vi "PPS Type Parser.vi"(5 "ClassName":string, 7 "Value":variant, 8 "error in (no error)":errorcluster, 10 "trimmed string":string, 11 "Control in":refnum<vi>) -> (0 "error out":errorcluster, 3 "spreadsheet string":string)   [LabVIEW 2016]
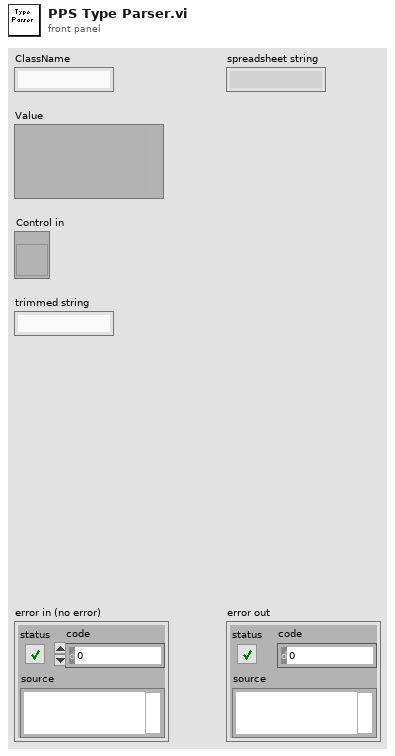
[diagram p1: front panel]
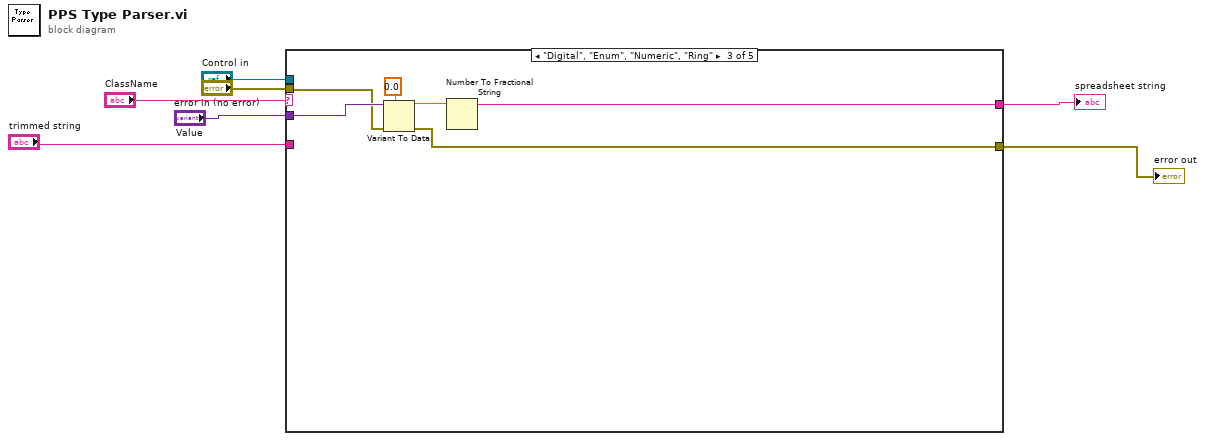
[diagram p0: block diagram]
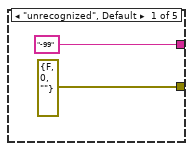
[diagram p2: hidden frame]
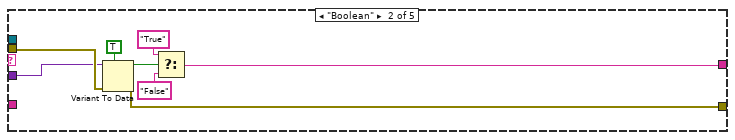
[diagram p3: hidden frame]
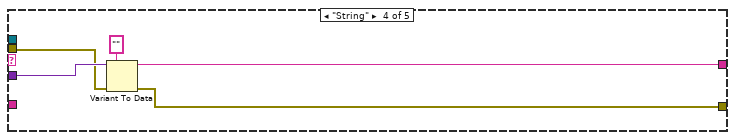
[diagram p4: hidden frame]
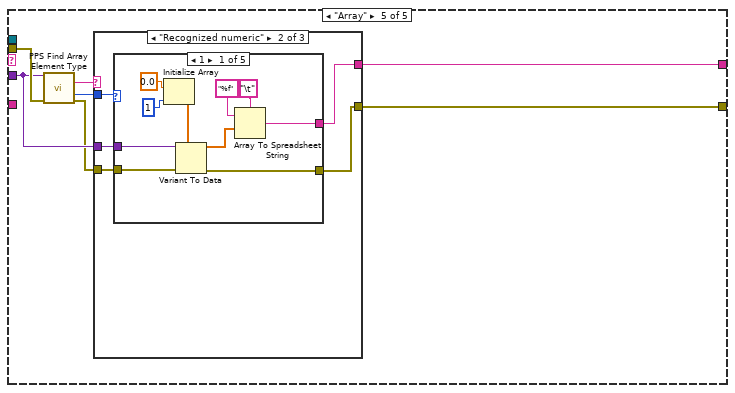
[diagram p5: hidden frame]
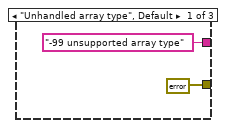
[diagram p6: hidden frame]
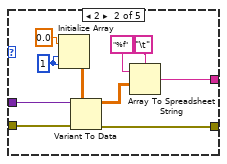
[diagram p7: hidden frame]
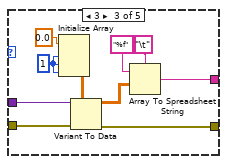
[diagram p8: hidden frame]
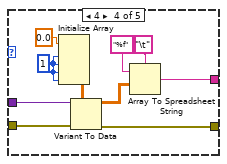
[diagram p9: hidden frame]
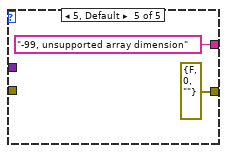
[diagram p10: hidden frame]
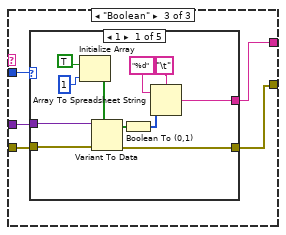
[diagram p11: hidden frame]
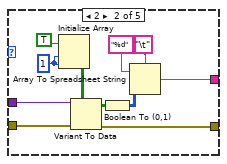
[diagram p12: hidden frame]
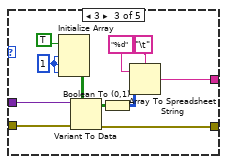
[diagram p13: hidden frame]
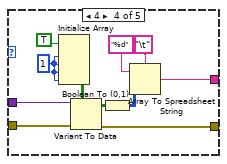
[diagram p14: hidden frame]
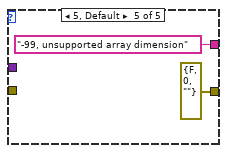
[diagram p15: hidden frame]
diagram:
  n1 = case shown="\"Digital\", \"Enum\", \"Numeric\", \"Ring\"" "ClassName" {
    tunnel: [errorcluster {"status"=FALSE, "code"=0, "source"=""} ("error out") w17 w23 w28 w31] -> w1
    tunnel: "Control in" -> [_ _ _ _ _]
    tunnel: "error in (no error)" -> [_ w11 w18 w24 w35]
    tunnel: ["-99" w12 w21 w27 w32] -> w5
    tunnel: "Value" -> [_ w10 w19 w25 w30]
    tunnel: "trimmed string" -> [_ _ _ _ _]
    frame "unrecognized", Default {
    }
    frame "Boolean" {
      n2 = Variant To Data(error in=w11, type=TRUE, Variant=w10) -> (data=w15:bool, error out=w17:errorcluster)
      n3 = Select(t="True", s=w15, f="False") -> (s? t:f=w12:string)
    }
    frame "Digital", "Enum", "Numeric", "Ring" {
      n4 = Variant To Data(error in=w18, type=0.0, Variant=w19) -> (data=w20:dbl, error out=w23:errorcluster)
      n5 = Number To Fractional String(number=w20) -> (F-format string=w21:string)  [unwired: 3 in]
    }
    frame "String" {
      n6 = Variant To Data(error in=w24, type="" ("data out"), Variant=w25) -> (data=w27:string, error out=w28:errorcluster)
    }
    frame "Array" {
      n7 = call "PPS Find Array Element Type.vi"("Variant"=w30, "error in (no error)"=w35) -> ("Element type Name"=w34:string, "Number of Dimensions"=w33:i32, "error out"=w29:errorcluster)  [unwired: 9 in, 2 out]
      n8 = case shown="\"Recognized numeric\"" w34 {
        tunnel: w33 -> [_ w42 w85]
        tunnel: ["-99 unsupported array type" ("spreadsheet string") w40 w86] -> w32
        tunnel: [errorcluster {"status"=FALSE, "code"=0, "source"=""} ("error out") w38 w87] -> w31
        tunnel: w30 -> [_ w41 w89]
        tunnel: w29 -> [_ w39 w88]
        frame "Unhandled array type", Default {
        }
        frame "Recognized numeric" {
          n9 = case shown="1" w42 {
            tunnel: w41 -> [w47 w58 w68 w78 _]
            tunnel: [w45 w56 w66 w76 "-99, unsupported array dimension" ("spreadsheet string")] -> w40
            tunnel: w39 -> [w44 w55 w65 w75 _]
            tunnel: [w43 w54 w64 w74 errorcluster {"status"=FALSE, "code"=0, "source"=""} ("error out")] -> w38
            frame 1 {
              n10 = Initialize Array(0.0 ("element"), 1 ("dimension size")) -> (w48:dbl[])
              n11 = Variant To Data(error in=w44, type=w48, Variant=w47) -> (data=w46:dbl[], error out=w43:errorcluster)
              n12 = Array To Spreadsheet String(delimiter (Tab)="\t", array=w46, 3:"%f" ("format string")) -> (spreadsheet string=w45:string)
            }
            frame 2 {
              w53 = 1 ("dimension size")
              n13 = Initialize Array(0.0 ("element"), w53, w53) -> (w59:dbl[][])
              n14 = Variant To Data(error in=w55, type=w59, Variant=w58) -> (data=w57:dbl[][], error out=w54:errorcluster)
              n15 = Array To Spreadsheet String(delimiter (Tab)="\t", array=w57, 3:"%f" ("format string")) -> (spreadsheet string=w56:string)
            }
            frame 3 {
              w63 = 1 ("dimension size")
              n16 = Initialize Array(0.0 ("element"), w63, w63, w63) -> (w69:dbl[][][])
              n17 = Variant To Data(error in=w65, type=w69, Variant=w68) -> (data=w67:dbl[][][], error out=w64:errorcluster)
              n18 = Array To Spreadsheet String(delimiter (Tab)="\t", array=w67, 3:"%f" ("format string")) -> (spreadsheet string=w66:string)
            }
            frame 4 {
              w73 = 1 ("dimension size")
              n19 = Initialize Array(0.0 ("element"), w73, w73, w73, w73) -> (w79:dbl[][][][])
              n20 = Variant To Data(error in=w75, type=w79, Variant=w78) -> (data=w77:dbl[][][][], error out=w74:errorcluster)
              n21 = Array To Spreadsheet String(delimiter (Tab)="\t", array=w77, 3:"%f" ("format string")) -> (spreadsheet string=w76:string)
            }
            frame 5, Default {
            }
          }
        }
        frame "Boolean" {
          n22 = case shown="1" w85 {
            tunnel: w89 -> [w96 w108 w119 w130 _]
            tunnel: [w95 w107 w118 w129 "-99, unsupported array dimension" ("spreadsheet string")] -> w86
            tunnel: w88 -> [w94 w106 w117 w128 _]
            tunnel: [w93 w105 w116 w127 errorcluster {"status"=FALSE, "code"=0, "source"=""} ("error out")] -> w87
            frame 1 {
              n23 = Initialize Array(TRUE, 1 ("dimension size")) -> (w97:bool[])
              n24 = Variant To Data(error in=w94, type=w97, Variant=w96) -> (data=w92:bool[], error out=w93:errorcluster)
              n25 = Boolean To (0,1)(Boolean=w92) -> (0, 1=w90:i16[])
              n26 = Array To Spreadsheet String(delimiter (Tab)="\t", array=w90, 3:"%d" ("format string")) -> (spreadsheet string=w95:string)
            }
            frame 2 {
              w101 = 1 ("dimension size")
              n27 = Initialize Array(TRUE, w101, w101) -> (w109:bool[][])
              n28 = Variant To Data(error in=w106, type=w109, Variant=w108) -> (data=w104:bool[][], error out=w105:errorcluster)
              n29 = Boolean To (0,1)(Boolean=w104) -> (0, 1=w102:i16[][])
              n30 = Array To Spreadsheet String(delimiter (Tab)="\t", array=w102, 3:"%d" ("format string")) -> (spreadsheet string=w107:string)
            }
            frame 3 {
              w112 = 1 ("dimension size")
              n31 = Initialize Array(TRUE, w112, w112, w112) -> (w120:bool[][][])
              n32 = Variant To Data(error in=w117, type=w120, Variant=w119) -> (data=w115:bool[][][], error out=w116:errorcluster)
              n33 = Boolean To (0,1)(Boolean=w115) -> (0, 1=w113:i16[][][])
              n34 = Array To Spreadsheet String(delimiter (Tab)="\t", array=w113, 3:"%d" ("format string")) -> (spreadsheet string=w118:string)
            }
            frame 4 {
              w123 = 1 ("dimension size")
              n35 = Initialize Array(TRUE, w123, w123, w123, w123) -> (w131:bool[][][][])
              n36 = Variant To Data(error in=w128, type=w131, Variant=w130) -> (data=w126:bool[][][][], error out=w127:errorcluster)
              n37 = Boolean To (0,1)(Boolean=w126) -> (0, 1=w124:i16[][][][])
              n38 = Array To Spreadsheet String(delimiter (Tab)="\t", array=w124, 3:"%d" ("format string")) -> (spreadsheet string=w129:string)
            }
            frame 5, Default {
            }
          }
        }
      }
    }
  }
  "spreadsheet string" <- w5
  "error out" <- w1
